vi "Validate Group Name.vi"(0 "Group Name in":string) -> (4 "Group Name out":string)   [LabVIEW 2021, in "InstrumentStudio Plug-In Editor.lvlib"]
uses:
  InstrumentStudio Plug-In Editor.lvlib
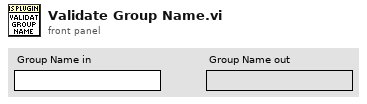
[diagram p1: front panel]
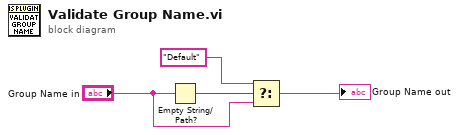
[diagram p0: block diagram]
diagram:
  n1 = Empty String/Path?(string/path="Group Name in") -> (empty?=w2:bool)
  n2 = Select(t="Default", s=w2, f="Group Name in") -> (s? t:f=→"Group Name out":string)
